vi "Enable Serial Input Channels New.vi"(0 "fpga interface in":refnum<k20>, 5 "serial input channels":string[](array[string]), 11 "error in (no error)":errorcluster) -> (4 "fpga interface out":refnum<k20>, 6 "channel configs":T1(array[cluster]), 8 "channel configs 2":T1(array[cluster]), 15 "error out":errorcluster)   [LabVIEW 2026]
uses:
  Types/148x_Acq_FPGA_Reference.ctl
  <instrlib>/FlexRIO/API/Host/v1/NI FlexRIO/API/Get Property Reference - Fpga Small.vi
  <vilib>/Utility/error.llb/Error Cluster From Error Code.vi
  <vilib>/rvi/errors/niLvFpgaAdjustHostInterfaceError.vi
  <vilib>/rvi/interface/nirviReadWriteControl/nirviReadWriteControl.xnode
  <resource>/objmgr/niflexrioapi.rc
  <instrlib>/FlexRIO/API/Host/v1/NI FlexRIO API v1.lvlib
  GettingStarted_Acq_148X_Host.lvlib
  NiFpgaLv.dll
  <vilib>/rvi/interface/Simulation/niFpgaSimulationCallBeginRW.vi
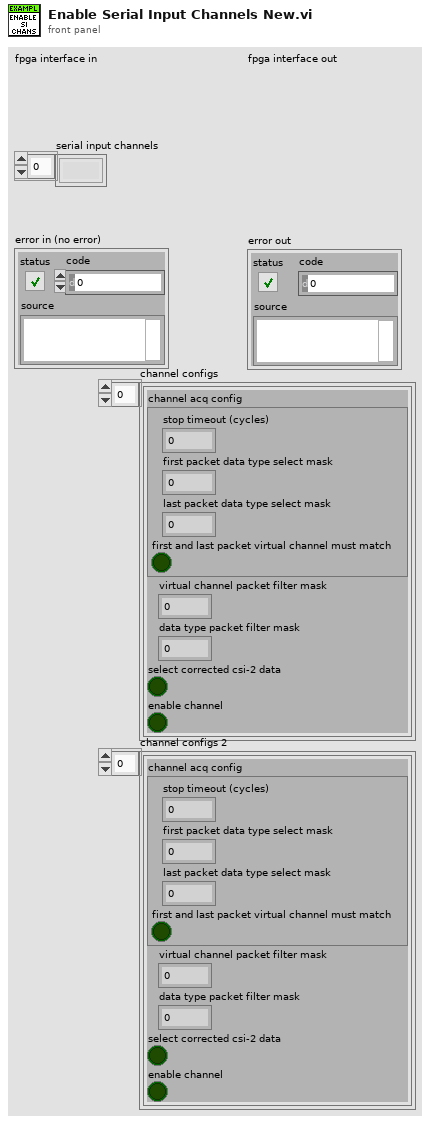
[diagram p1: front panel]
types:
  T1 = cluster{"channel acq config":cluster{"stop timeout (cycles)":u32, "first packet data type select mask":u64, "last packet data type select mask":u64, "first and last packet virtual channel must match":bool}, "virtual channel packet filter mask":u16, "data type packet filter mask":u64, "select corrected csi-2 data":bool, "enable channel":bool}[]
  T2 = typedef "GettingStarted_Acq_148X_Host.lvlib/148x_Acq_FPGA_Reference.ctl" = refnum<k20>
  T3 = cluster{"channel acq config":cluster{"stop timeout (cycles)":u32, "first packet data type select mask":u64, "last packet data type select mask":u64, "first and last packet virtual channel must match":bool}, "virtual channel packet filter mask":u16, "data type packet filter mask":u64, "select corrected csi-2 data":bool, "enable channel":bool}
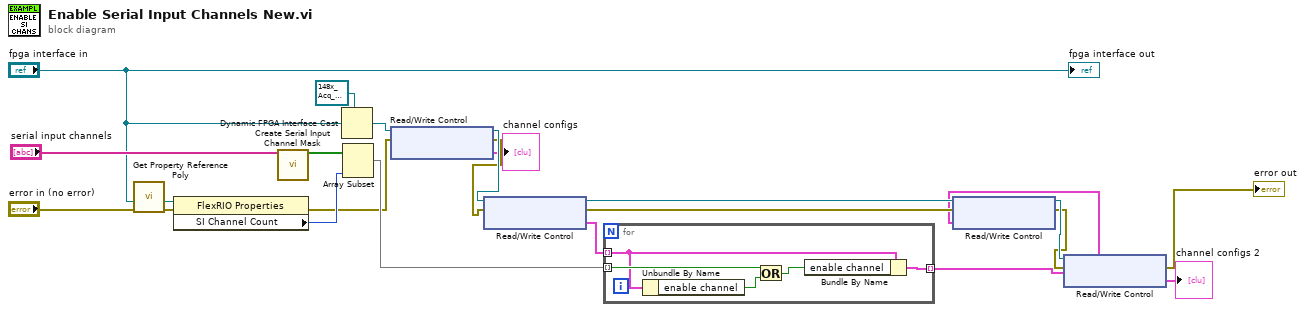
[diagram p0: block diagram]
diagram:
  n1 = call-poly <instrlib>:"Get Property Reference Poly.vi"("error in (no error)"="error in (no error)", "fpga interface in"="fpga interface in") -> ("error out"=w20:errorcluster, "property reference"=w21:refnum<k20>)  [unwired: 4 in, 1 out]
  n2 = property class="FlexRIO Properties"(reference=w21, error in=w20) -> (error out=w8:errorcluster, "SI Channel Count"=w15:i32)  [unwired: 1 out]
  n3 = call "Create Serial Input Channel Mask.vi"("serial channels"="serial input channels") -> ("serial input channel mask"=w17:bool[])  [unwired: 14 in]
  n4 = Dynamic FPGA Interface Cast(Session In=T2 refnum ("FPGA VI Reference Out"), Type="fpga interface in") -> (Session Out=w9:T2)
  n5 = Array Subset(array=w17, length=w15) -> (w13:bool[])  [unwired: 1 in]
  n6 = xnode "Read/Write Control"("FPGA VI Reference In"=w9, "error in"=w8) -> ("FPGA VI Reference Out"=w7:T2, "error out"=w6:errorcluster, "channel configs"=→"channel configs":T1)
  n7 = xnode "Read/Write Control"("FPGA VI Reference In"=w7, "error in"=w6) -> ("FPGA VI Reference Out"=w11:T2, "error out"=w12:errorcluster, "channel configs"=w14:T1)
  n8 = for {
    tunnel: w14 -> [w25] mode=indexing
    tunnel: w13 -> [w27] mode=indexing
    tunnel: [w26] -> w10 mode=indexing
    n9 = Unbundle By Name(w25) -> ("enable channel"=w23:bool)
    n10 = Or(x=w27, y=w23) -> (x .or. y?=w24:bool)
    n11 = Bundle By Name(cluster=w25, "enable channel"=w24) -> (w26:T3)
  }
  n12 = xnode "Read/Write Control"("FPGA VI Reference In"=w11, "error in"=w12, "channel configs"=w10) -> ("FPGA VI Reference Out"=w3:T2, "error out"=w2:errorcluster)
  n13 = xnode "Read/Write Control"("FPGA VI Reference In"=w3, "error in"=w2) -> ("error out"=→"error out":errorcluster, "channel configs"=→"channel configs 2":T1)  [unwired: 1 out]
  "fpga interface out" <- "fpga interface in"
